vi "Get Integer Variable.vi"(8 "error in (no error)":errorcluster, 10 "Name":string, 11 "Application in":refnum<class "Application.lvclass">) -> (0 "error out":errorcluster, 2 "Value":i64, 3 "Application out":refnum<class "Application.lvclass">)   [LabVIEW 2017, in "Application.lvlib" / "Application.lvclass"]
doc: "Retrieves a named variable from the local variable engine and casts it as a integer."
uses:
  Application.lvclass
  <vilib>/TSS/ACRObat Test Framework/Classes/Variable Engine/Class/Variable Engine.lvclass
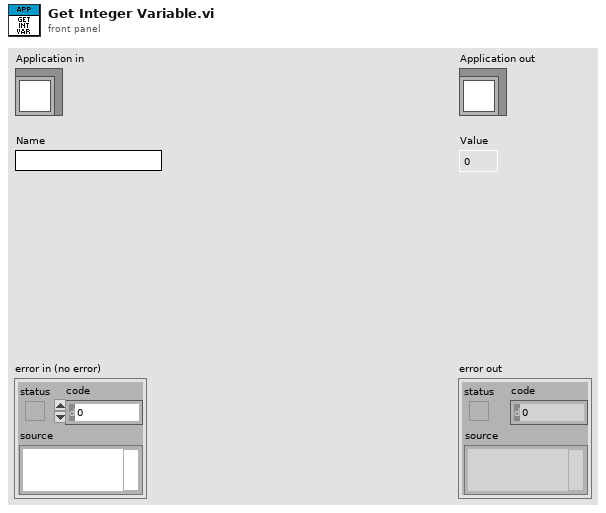
[diagram p1: front panel]
types:
  T1 = typedef "Application.lvlib/App Properties.lvclass/Class Properties -- Cluster.ctl" = cluster{"UUT Info":T2[], "Test Information":refnum<vi>, "Gold Board":refnum<class "Golden Board.lvclass">, "Test Recipe":refnum<class "Test Recipe.lvclass">, "Instruments":refnum<class "Instrument.lvclass">[], "Mode":T3, "Test Results":T4[], "Station Config":refnum<class "Station Config.lvclass">, "Variable Engine":refnum<class "Variable Engine.lvclass">}
  T2 = typedef "Application.lvlib/App Properties.lvclass/UUT Reference -- Cluster.ctl" = cluster{"Serial Number Reference":refnum<vi>, "Status Message Reference":refnum<vi>}
  T3 = typedef "Application.lvlib/Application.lvclass/Op Mode -- Enum.ctl" = u16
  T4 = typedef "Application.lvlib/App Properties.lvclass/Test Result -- Cluster.ctl" = cluster{"Position":i32, "Pass":bool, "Fail Codes":string}
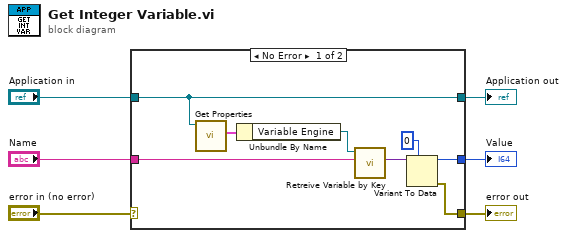
[diagram p0: block diagram]
diagram:
  n1 = case shown="No Error" "error in (no error)" {
    selector: "error in (no error)" -> [_ w16]
    tunnel: [w8 w16] -> w5
    tunnel: [w11 w15] -> w3
    tunnel: "Application in" -> [w11 w15]
    tunnel: "Name" -> [w13 _]
    tunnel: [w12 _] -> w1
    frame No Error {
      n2 = call "Get Properties.vi"("Acrobat Template in"=w11) -> ("Class Properties"=w10:T1)  [unwired: 8 in, 2 out]
      n3 = Unbundle By Name(w10) -> ("Variable Engine"=w9:refnum<class "Variable Engine.lvclass">)
      n4 = call <vilib>:"Retreive Variable by Key.vi"("Key"=w13, "Acrobat Template in"=w9) -> ("Value"=w14:variant)  [unwired: 7 in, 2 out]
      n5 = Variant To Data(type=i64 0 ("Value"), Variant=w14) -> (data=w12:i64, error out=w8:errorcluster)  [unwired: 1 in]
    }
    frame Error {
    }
  }
  "error out" <- w5
  "Application out" <- w3
  "Value" <- w1
